vi "Cell release.vi"(11 "EV3 in":T1) -> (2 "Ini. Degrees":sgl, 3 "EV3 out":T1)   [LabVIEW 2016]
uses:
  <vilib>/NXT/Subs/LVHSConnector.ctl
  <vilib>/NXT/LegoClasses/BrickReference/BrickReference.lvclass
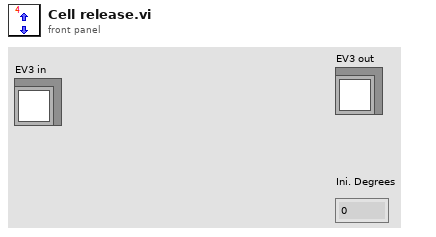
[diagram p1: front panel]
types:
  T1 = typedef "LVHSConnector.ctl" = refnum<class "BrickReference.lvclass">
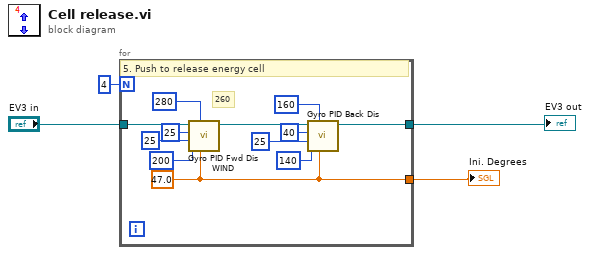
[diagram p0: block diagram]
diagram:
  n1 = for {
    N: 4 -> [_]
    tunnel: [w8] -> w4
    tunnel: [w7] -> w2
    tunnel: "EV3 in" -> [w5]
    w7 = sgl 47.0 ("Ini. Degrees")
    # "260"
    # "5. Push to release energy cell"
    n2 = call "Gyro PID Fwd Dis WIND.vi"("Target angle"=w7, "Threshold to stop"=280 ("Stop rotation"), "Threshold to slow"=200 ("Threshold to De-acc"), "Higher speed"=25 ("De-acc"), "Max. speed"=25 ("Acc"), "EV3 in"=w5) -> ("EV3 out"=w9:T1)  [unwired: 5 in]
    n3 = call "Gyro PID Back Dis.vi"("Target angle"=w7, "Threshold to stop"=160 ("Stop rotation"), "Threshold to slow"=140 ("Threshold to De-acc"), "Min. speed"=25 ("De-acc"), "Max. speed"=40 ("Acc"), "EV3 in"=w9) -> ("EV3 out"=w8:T1)  [unwired: 5 in]
  }
  "EV3 out" <- w4
  "Ini. Degrees" <- w2
